vi "Convert RF Power to Array.vi"(8 "error in (no error)":errorcluster, 11 "ModSweep in":refnum<class "Power Sweep.lvclass">) -> (0 "error out":errorcluster, 3 "ModSweep out":refnum<class "Power Sweep.lvclass">)   [LabVIEW 2018, in "Power Sweep.lvlib" / "Power Sweep.lvclass"]
uses:
  Power Sweep.lvclass
  C:/Sequence Automation/Plugins/Measurement Interface.lvlibp/Measurement Interface.lvclass
  Power Sweep.lvclass/Power Sweep.ctl
  Plugins/Measurement Interface.lvlibp/Private Methods/Measurement Parameters/Read Measurement Parameters.vi
  Plugins/String Database.lvlibp/String Database.lvclass
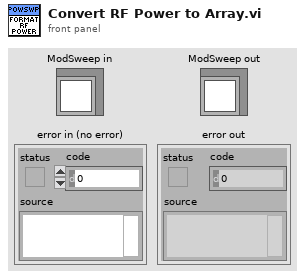
[diagram p1: front panel]
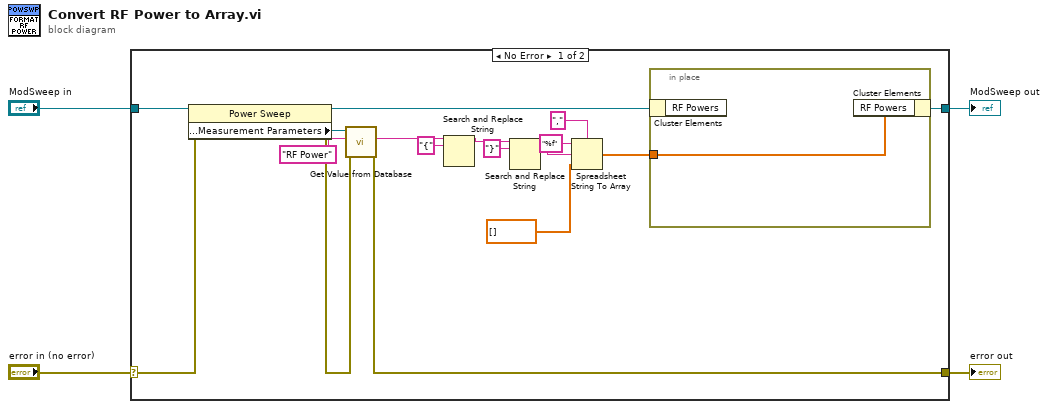
[diagram p0: block diagram]
diagram:
  n1 = case shown="No Error" "error in (no error)" {
    selector: "error in (no error)" -> [w21 w24]
    tunnel: [w18 w24] -> w3
    tunnel: [w6 w23] -> w1
    tunnel: "ModSweep in" -> [w20 w23]
    frame No Error {
      n2 = property class="Power Sweep"(reference=w20, error in=w21) -> (reference out=w8:refnum<class "Power Sweep.lvclass">, error out=w19:errorcluster, "Protected Methods:Measurement Parameters"=w17:refnum<class "String Database.lvclass">)
      n3 = call "Get Value from Database.vi"("error in (no error)"=w19, "Entry Name"="RF Power", "Message in"=w17) -> ("error out"=w18:errorcluster, "Entry Value"=w15:string)  [unwired: 5 in, 2 out]
      n4 = Search and Replace String(input string=w15, search string="{") -> (result string=w13:string)  [unwired: 6 in, 3 out]
      n5 = Search and Replace String(input string=w13, search string="}") -> (result string=w11:string)  [unwired: 6 in, 3 out]
      n6 = Spreadsheet String To Array(delimiter (Tab)=",", format string="%f", spreadsheet string=w11, array type (2D Dbl)=dbl[] []) -> (array=w7:dbl[])
      n7 = in-place {
        in-place-border: w7 -> [w22]
        n8 = in-place-cluster #1(w8) -> ()  [unwired: 1 out]
        n9 = in-place-cluster #1("RF Powers"=w22) -> (w6:refnum<class "Power Sweep.lvclass">)
      }
    }
    frame Error {
    }
  }
  "error out" <- w3
  "ModSweep out" <- w1
